vi "DMA.Scatter-Gather.Get Transfer Size.vi"(11 "Scatter-Gather Transfer Spec":T1 {"Block Descriptors"."next descriptor ptr" format="%08x"; "Block Descriptors"."data size" format="%08x"; "Block Descriptors"."data ptr (upper)" format="%08x"; "Block Descriptors"."data ptr (lower)" format="%08x"; "Block Descriptors"."descriptor ptr (aligned)" format="%08x"; "Block Descriptors"."descriptor size" format="%08x"; "Block Descriptors"."descriptor ptr (VISA)" format="%08x"; "RFM Address" format="%08x"}) -> (2 "Transfer Size (bytes)":u32, 3 "Scatter-Gather Transfer Spec out":T1 {"Block Descriptors"."next descriptor ptr" format="%08x"; "Block Descriptors"."data size" format="%08x"; "Block Descriptors"."data ptr (upper)" format="%08x"; "Block Descriptors"."data ptr (lower)" format="%08x"; "Block Descriptors"."descriptor ptr (aligned)" format="%08x"; "Block Descriptors"."descriptor size" format="%08x"; "Block Descriptors"."descriptor ptr (VISA)" format="%08x"; "RFM Address" format="%08x"})   [LabVIEW 2016, in "GE 5565PIORC.lvclass"]
uses:
  GE 5565PIORC.lvclass
  Controls/DMA Transfer Spec (Scatter-Gather).ctl
  Controls/DMA Block Descriptor.ctl
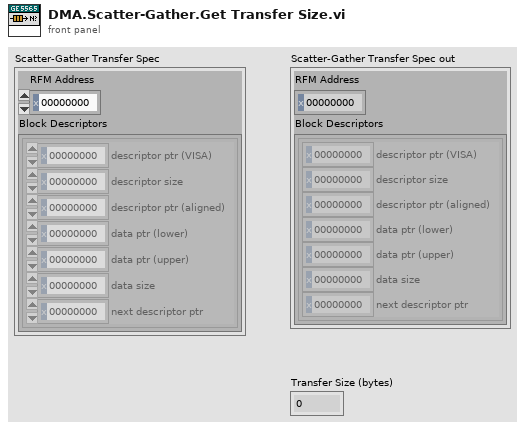
[diagram p1: front panel]
types:
  T1 = typedef "GE 5565PIORC.lvclass/DMA Transfer Spec (Scatter-Gather).ctl" = cluster{"RFM Address":u32, "Block Descriptors":T2[]}
  T2 = typedef "GE 5565PIORC.lvclass/DMA Block Descriptor.ctl" = cluster{"descriptor ptr (VISA)":u32, "descriptor size":u32, "descriptor ptr (aligned)":u32, "data ptr (lower)":u32, "data ptr (upper)":u32, "data size":u32, "next descriptor ptr":u32}
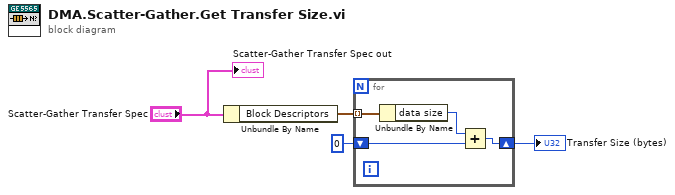
[diagram p0: block diagram]
diagram:
  n1 = Unbundle By Name("Scatter-Gather Transfer Spec") -> ("Block Descriptors"=w2:T2[])
  n2 = for {
    tunnel: w2 -> [w8] mode=indexing
    shift-right: [w5] -> w3
    shift-left: u32 0 -> [w6]
    n3 = Unbundle By Name(w8) -> ("data size"=w7:u32)
    n4 = Add(x=w7, y=w6) -> (x+y=w5:u32)
  }
  "Transfer Size (bytes)" <- w3
  "Scatter-Gather Transfer Spec out" <- "Scatter-Gather Transfer Spec"
